vi "CurrentAngle.vi"(9 "Theta":dbl, 10 "Beta":dbl, 11 "Alpha":dbl) -> (2 "Current Angle":dbl)   [LabVIEW 2014]
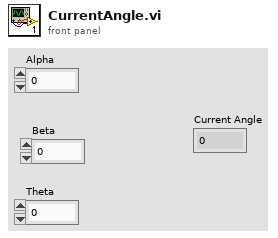
[diagram p1: front panel]
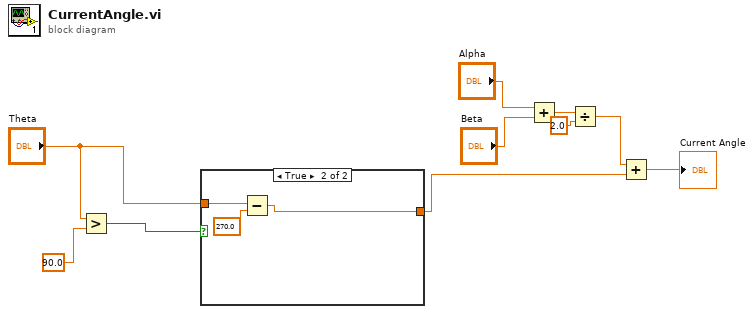
[diagram p0: block diagram]
diagram:
  n1 = Greater?(x="Theta", y=90.0) -> (0:w3:bool)
  n2 = case shown="True" w3 {
    tunnel: "Theta" -> [w11 w14]
    tunnel: [w11 w12] -> w1
    frame False {
    }
    frame True {
      n3 = Subtract(x=w14, y=270.0) -> (x-y=w12:dbl)
    }
  }
  n4 = Add(x="Alpha", y="Beta") -> (x+y=w8:dbl)
  n5 = Divide(x=w8, y=2.0) -> (x/y=w6:dbl)
  n6 = Add(x=w6, y=w1) -> (x+y=→"Current Angle":dbl)
